vi "State_Machine.vi"(8 "error in (no error)":errorcluster caption="entrée d'erreur (pas d'erreur)", 11 "Flash_Jlink en entrée":refnum<class "FW_Check_Hash_code.lvclass">) -> (0 "error out":errorcluster caption="sortie d'erreur", 2 "Json_String":string, 3 "Flash_Jlink en sortie":refnum<class "FW_Check_Hash_code.lvclass">)   [LabVIEW 2020, in "Library Test.lvlib" / "FW_Check_Hash_code.lvclass"]
uses:
  FW_Check_Hash_code.lvclass
  Cryptographic Hash/Cryptographic Hash_SHA256_File/Cryptographic Hash_SHA256_File.lvclass
  C:/Users/ngarcin/OneDrive - Altyor/Standard TB/Class/Cryptographic Hash/Cryptographic Hash (Default)/Cryptographic Hash (Default).lvclass
  FW_Check_Hash_code.lvclass/FW_Check_Hash_code.ctl
panel:
  out "String In progress":string
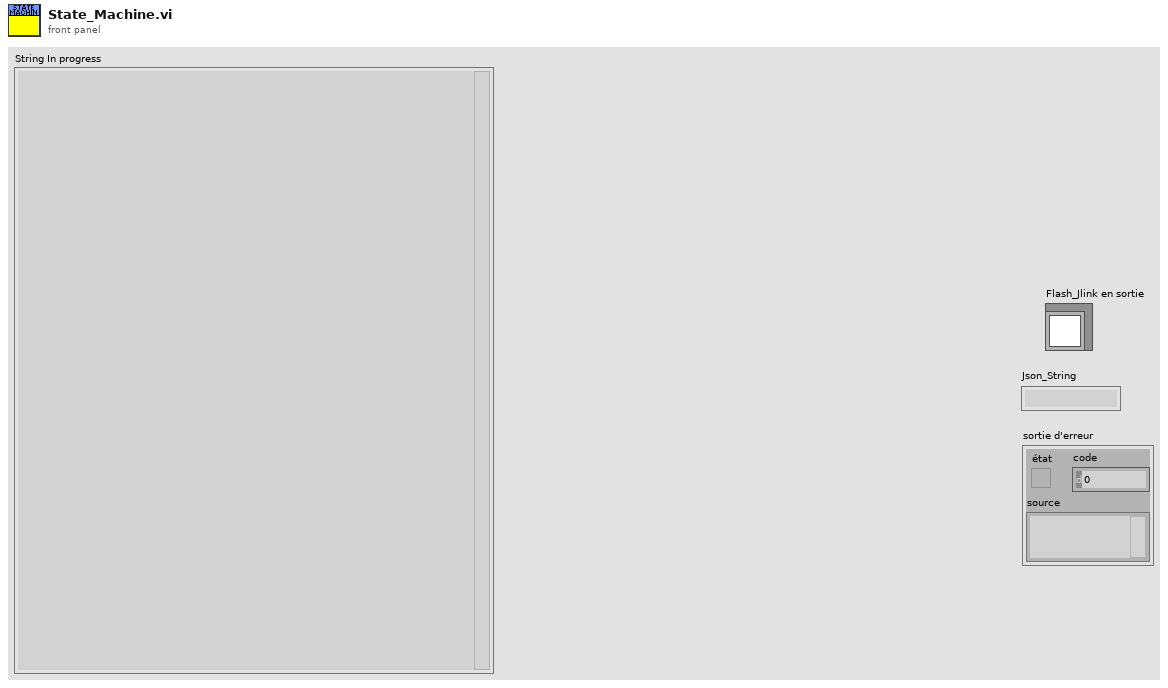
[diagram p1: front panel]
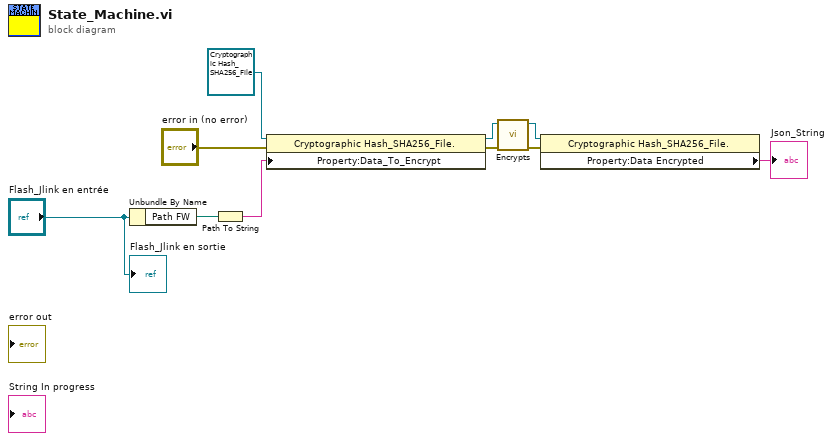
[diagram p0: block diagram]
diagram:
  n1 = Unbundle By Name("Flash_Jlink en entrée") -> ("Path FW"=w3:path)
  n2 = Path To String(path=w3) -> (string=w2:string)
  n3 = property class="Cryptographic Hash_SHA256_File."(reference=refnum<class "Cryptographic Hash_SHA256_File.lvclass"> refnum ("Library Cryptographic Hash.lvlib:Cryptographic Hash_SHA256_File.lvclass"), error in="error in (no error)", "Property:Data_To_Encrypt"=w2) -> (reference out=w9:refnum<class "Cryptographic Hash_SHA256_File.lvclass">, error out=w6:errorcluster)
  n4 = call-dynamic "Encrypts.vi"("error in (no error)"=w6, "Cryptographic Hash_SHA256 en entrée"=w9) -> ("error out"=w7:errorcluster, "Cryptographic Hash_SHA256 en sortie"=w8:refnum<class "Cryptographic Hash_SHA256_File.lvclass">)  [unwired: 8 in]
  n5 = property class="Cryptographic Hash_SHA256_File."(reference=w8, error in=w7) -> ("Property:Data Encrypted"=→"Json_String":string)  [unwired: 2 out]
  "Flash_Jlink en sortie" <- "Flash_Jlink en entrée"
